vi "Read from File.vi"(11 "Config name":string) -> (3 "Devices":refnum<class "Device.lvclass">[](array[class]))   [LabVIEW 2019, in "SLMP.lvlib" / "Device.lvclass"]
uses:
  Device.lvclass
  Device.lvclass/Device.ctl
  b267523d-e4f6-4961-9193-903b803d71cc.vi
  9fa35442-2741-41ad-bfe8-1f1194858088.vi
  <vilib>/JDP Science/JSONtext/Find Item.vi
  <vilib>/JDP Science/JSONtext/String Subset.vi
  <vilib>/JDP Science/JSONtext/Parsing/Parse Full Path or Item Name.vi
  <vilib>/JDP Science/JSONtext/Next JSON Value.vi
  <vilib>/JDP Science/JSONtext/support/Error Cluster From Code.vi
  <vilib>/JDP Science/JSONtext/Offset/Find Item Locations by Path.vi
  <vilib>/JDP Science/JSONtext/JSON text to Variant.vi
  <vilib>/JDP Science/JSONtext/Variant to JSON Text.vi
  <vilib>/JDP Science/JSONtext/LVClass Serializer/JSONtext LVClass Serializer.lvclass
  SLMP.lvlib
  <vilib>/JDP Science/JSONtext/JSONtext.lvlib
panel:
  out "Updated devices":string[](array[string])
  out "text":string
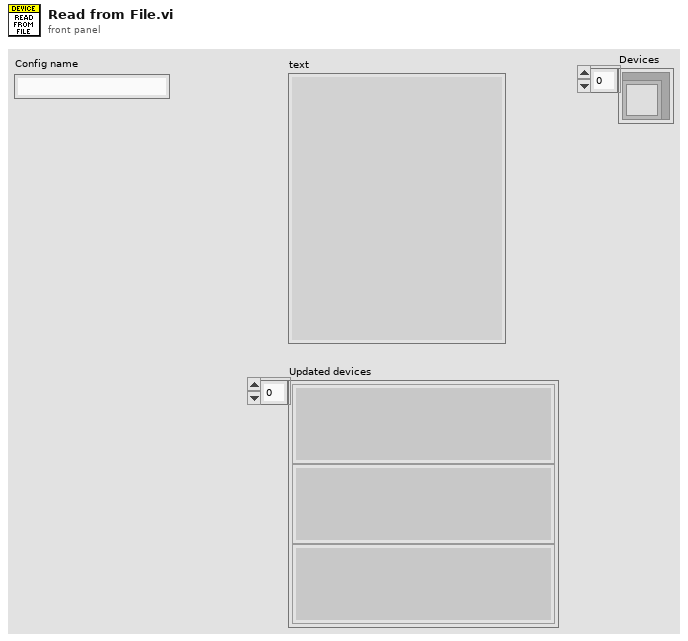
[diagram p1: front panel]
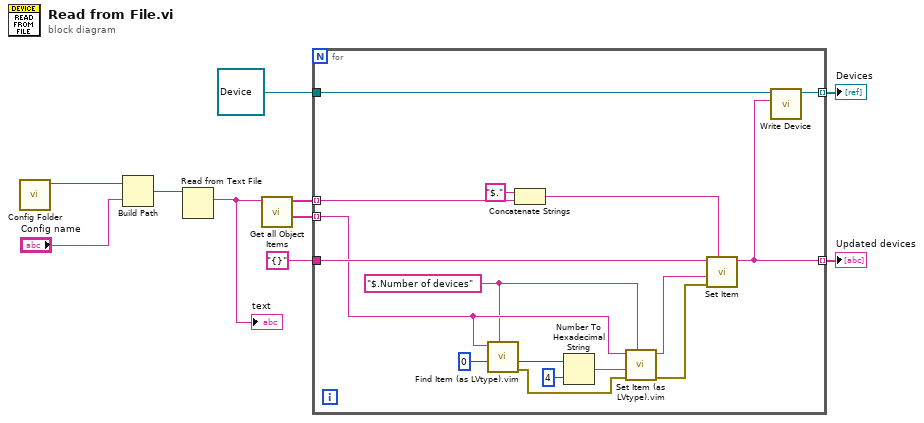
[diagram p0: block diagram]
diagram:
  n1 = call "Config Folder.vi"() -> (".config folder"=w10:path)  [unwired: 11 in]
  n2 = Build Path(base path=w10, name or relative path="Config name") -> (appended path=w9:path)
  n3 = Read from Text File(file (use dialog)=w9) -> (text=w8:string)  [unwired: 3 in, 3 out]
  "text" <- w8
  n4 = call <vilib>:"Get all Object Items.vi"("JSON"=w8) -> ("<JSON>"=w6:string[], "Item Names"=w7:string[])  [unwired: 7 in, 2 out]
  n5 = for {
    tunnel: w7 -> [w25] mode=indexing
    tunnel: w6 -> [w18] mode=indexing
    tunnel: refnum<class "Device.lvclass"> refnum ("SLMP.lvlib:Device.lvclass") -> [w13]
    tunnel: "{}" -> [w26]
    tunnel: [w12] -> w3 mode=indexing
    tunnel: [w11] -> w2 mode=indexing
    w17 = "$.Number of devices" ("$Path or Item Name")
    n6 = call "Find Item (as LVtype).vim"("$Path or Item Name"=w17, "Data Type and Default Value"=0, "JSON"=w18) -> ("error out"=w14:errorcluster, "Data"=w21:i32)  [unwired: 5 in, 2 out]
    n7 = Concatenate Strings("$." ("string"), w25) -> (w23:string)
    n8 = Number To Hexadecimal String(1:i16 4 ("width (-)"), 2:w21) -> (0:w19:string)
    n9 = call "Set Item (as LVtype).vim"("Object (or Item) Path"=w17, "error in (no error)"=w14, "Anything"=w19, "JSON"=w18) -> ("error out"=w15:errorcluster, "<JSON>"=w16:string)  [unwired: 4 in, 1 out]
    n10 = call <vilib>:"Set Item.vi"("$Path or Item Name"=w23, "error in (no error)"=w15, "JSON to Insert"=w16, "JSON"=w26) -> ("<JSON>"=w12:string)  [unwired: 4 in, 2 out]
    n11 = call "Write Device.vi"("Device"=w12, "Device in"=w13) -> ("Device out"=w11:refnum<class "Device.lvclass">)  [unwired: 8 in, 1 out]
  }
  "Updated devices" <- w3
  "Devices" <- w2
